vi "merFISH_set_autofocus_to_ref_position.vi"(5 "queue ASI stage":refnum<queue>, 7 "queue piezo":refnum<queue>, 8 "error in":errorcluster, 10 "Ref":dbl) -> (0 "error out":errorcluster)   [LabVIEW 2015]
uses:
  CONTROLS/Q_ASI_stage_element.ctl
  CONTROLS/Q_MCL_piezo_element.ctl
  GLOBAL/Global_MCL_piezo.vi
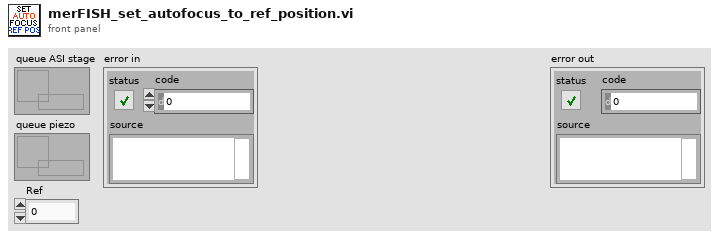
[diagram p1: front panel]
types:
  T1 = typedef "Q_MCL_piezo_element.ctl" = cluster{"variant":variant, "Instruction":enum16{"Piezo_idle", "Piezo_initialize", "Piezo_error", "Piezo_security_stop", "Piezo_read_z", "Piezo_move_z", "Piezo_keyboard_move", "Piezo_close_autofocus_calibration_ramp", "Piezo_change_init_state", "Piezo_init_autofocus", "Piezo_init_autofocus_merFISH_TL", "Piezo_autofocus", "Piezo_autofocus_merFISH_TL", "Piezo_stop_autofocus", "Piezo_stop_autofocus_merFISH_TL", "Piezo_autofocus_lost", "Piezo_resume_autofocus_merFISH_TL", "Piezo_check_z_position_merFISH_TL", "Piezo_init_ramp", "Piezo_move_z_ramp", "Piezo_close_ramp", "Piezo_close_merFISH", "Piezo_stop"}}
  T2 = typedef "Q_ASI_stage_element.ctl" = cluster{"variant":variant, "Instruction":enum16{"ASI_idle", "ASI_initialize", "ASI_error", "ASI_security_stop", "ASI_read_XYZ", "ASI_up", "ASI_down", "ASI_left", "ASI_right", "ASI_save_XY", "ASI_move_to_XY", "ASI_brightfield", "ASI_init_scan", "ASI_init_merFISH", "ASI_move_to_XY_merFISH", "ASI_move_to_Z_merFISH", "ASI_init_autofocus_search_merFISH", "ASI_close_autofocus_search_merFISH", "ASI_adjust_piezo_autofocus_merFISH", "ASI_set_piezo_autofocus_to_reference_position_merFISH_TL", "ASI_close_merFISH", "ASI_stop"}}
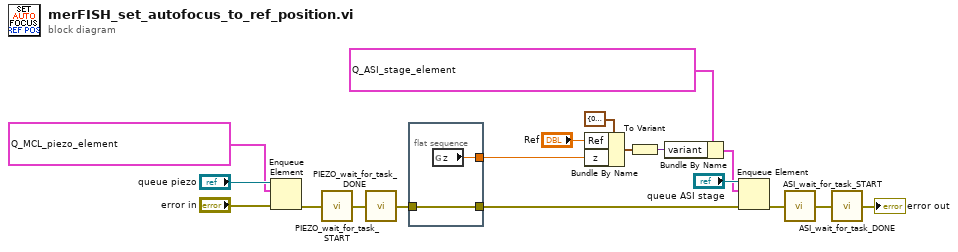
[diagram p0: block diagram]
diagram:
  n1 = Enqueue Element(queue="queue piezo", element=T1 {"variant"=variant, "Instruction"=enum."Piezo_check_z_position_merFISH_TL"}, error in (no error)="error in") -> (error out=w11:errorcluster)  [unwired: 1 in, 2 out]
  n2 = call "PIEZO_wait_for_task_START.vi"("error in"=w11) -> ("error out"=w10:errorcluster)
  n3 = call "PIEZO_wait_for_task_DONE.vi"("error in"=w10) -> ("error out"=w9:errorcluster)
  n4 = flat-sequence {
    tunnel: w9 -> [w20]
    tunnel: [w20] -> w7
    tunnel: [w19] -> w8
    frame #0 {
      n5 = global read "Global_MCL_piezo.vi" "z"() -> (w19:dbl)
    }
  }
  n6 = Bundle By Name(cluster=cluster{"Ref":dbl, "z":dbl} {"Ref"=0.0, "z"=0.0} ("Limits"), "Ref"="Ref", "z"=w8) -> (w14:cluster{"Ref":dbl, "z":dbl})
  n7 = To Variant(anything=w14) -> (Variant=w2:variant)
  n8 = Bundle By Name(cluster=T2 {"variant"=variant, "Instruction"=enum."ASI_set_piezo_autofocus_to_reference_position_merFISH_TL"} ("element"), "variant"=w2) -> (w16:T2)
  n9 = Enqueue Element(queue="queue ASI stage", element=w16, error in (no error)=w7) -> (error out=w5:errorcluster)  [unwired: 1 in, 2 out]
  n10 = call "ASI_wait_for_task_START.vi"("error in"=w5) -> ("error out"=w4:errorcluster)
  n11 = call "ASI_wait_for_task_DONE.vi"("error in"=w4) -> ("error out"=→"error out":errorcluster)
